vi "MSEditor_SaveMethodFile.vi"(8 "error in (no error)":errorcluster, 11 "Mthd in":T1) -> (0 "error out":errorcluster)   [LabVIEW 2018]
uses:
  Constant/AccessFolderName.ctl
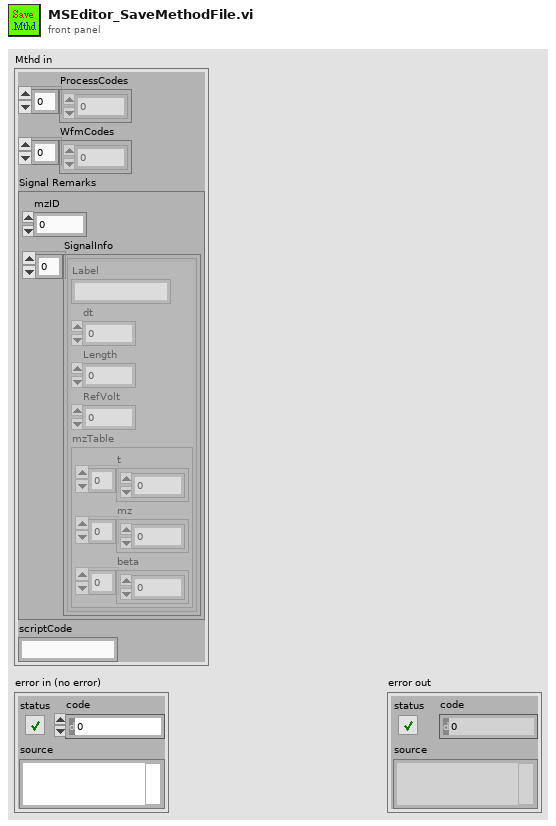
[diagram p1: front panel]
types:
  T1 = cluster{"ProcessCodes":u64[], "WfmCodes":u64[], "Signal Remarks":cluster{"mzID":u64, "SignalInfo":cluster{"Label":string, "dt":dbl, "Length":u32, "RefVolt":dbl, "mzTable":cluster{"t":dbl[], "mz":dbl[], "beta":dbl[]}}[]}, "scriptCode":string}
  T2 = typedef "AccessFolderName.ctl" = enum16{"None", "system_log", "ui_log", "msdata", "method", "d999_param"}
  T3 = enum16{"open", "replace", "create", "open or create", "replace or create", "replace or create with confirmation"}
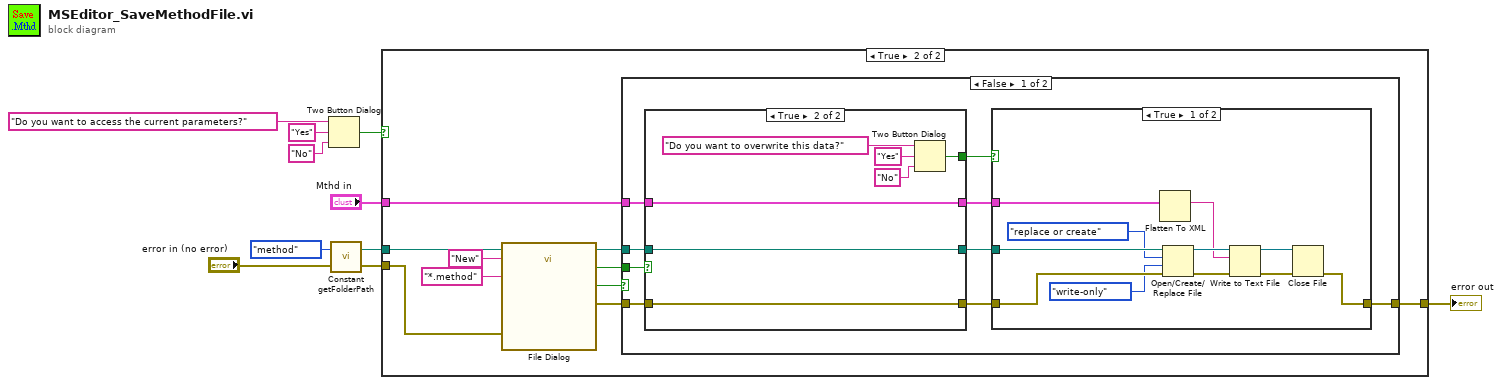
[diagram p0: block diagram]
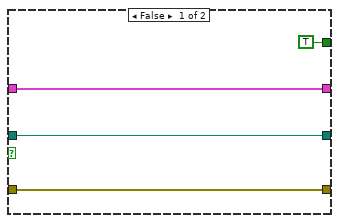
[diagram p4: hidden frame]
diagram:
  n1 = Two Button Dialog(message="Do you want to access the current parameters?", 1:"No" ("F button name (\"Cancel\")"), 2:"Yes" ("T button name (\"OK\")")) -> (T button?=w7:bool)
  n2 = call "Constant getFolderPath.vi"("error in (no error)"="error in (no error)", "folder name"=AccessFolderName."method") -> ("error out"=w2:errorcluster, "folder path"=w3:path)
  n3 = case shown="True" w7 {
    tunnel: [w11 w12] -> w6
    tunnel: w3 -> [_ w19]
    tunnel: w2 -> [w11 w18]
    tunnel: "Mthd in" -> [_ w16]
    frame False {
    }
    frame True {
      n4 = call "File Dialog"("start path"=w19, "default name"="New", "error in"=w18, "pattern (all files)"="*.method") -> ("selected path"=w15:path, "exists"=w13:bool, "cancelled"=w17:bool, "error out"=w14:errorcluster)  [unwired: 8 in]
      n5 = case shown="False" w17 {
        tunnel: w16 -> [w30 _]
        tunnel: w15 -> [w29 _]
        tunnel: w14 -> [w28 w54]
        tunnel: w13 -> [w27 _]
        tunnel: [w26 w54] -> w12
        frame False {
          n6 = case shown="True" w27 {
            tunnel: w30 -> [w44 w49]
            tunnel: w29 -> [w45 w48]
            tunnel: w28 -> [w46 w47]
            tunnel: [TRUE ("T button?") w50] -> w24
            tunnel: [w44 w49] -> w23
            tunnel: [w45 w48] -> w22
            tunnel: [w46 w47] -> w25
            frame False {
            }
            frame True {
              n7 = Two Button Dialog(message="Do you want to overwrite this data?", 1:"No" ("F button name (\"Cancel\")"), 2:"Yes" ("T button name (\"OK\")")) -> (T button?=w50:bool)
            }
          }
          n8 = case shown="True" w24 {
            tunnel: [w35 w42] -> w26
            tunnel: w25 -> [w40 w42]
            tunnel: w23 -> [w32 _]
            tunnel: w22 -> [w41 _]
            frame True {
              n9 = Flatten To XML(anything=w32) -> (xml string=w31:string)
              n10 = Open/Create/Replace File(file path (use dialog)=w41, error in=w40, operation (0:open)=T3."replace or create", access (0:read/write)=enum16{"read/write", "read-only", "write-only"}."write-only") -> (refnum out=w39:refnum<file>, error out=w38:errorcluster)  [unwired: 2 in, 1 out]
              n11 = Write to Text File(file (use dialog)=w39, text=w31, error in=w38) -> (refnum out=w37:refnum<file>, error out=w36:errorcluster)  [unwired: 1 in, 1 out]
              n12 = Close File(refnum=w37, error in=w36) -> (error out=w35:errorcluster)  [unwired: 1 out]
            }
            frame False {
            }
          }
        }
        frame True {
        }
      }
    }
  }
  "error out" <- w6
